vi "Get Block.vi"(8 "error in (no error)":errorcluster, 9 "Remove LenSize? (T)":bool=TRUE, 10 "Block Name":string, 11 "Content in":T2) -> (0 "error out":errorcluster, 1 "Block out":T1, 2 "Data out":string, 3 "Content out":T2, 4 "Found?":bool)   [LabVIEW 2018, in "VI-Hacker.lvlib"]
uses:
  VI-Hacker.lvlib
  TypeDefs/Block.ctl
  TypeDefs/Content.ctl
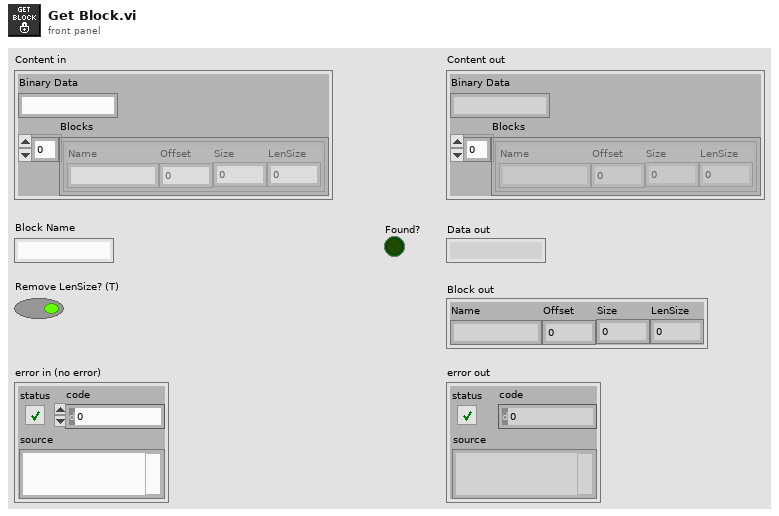
[diagram p1: front panel]
types:
  T1 = typedef "VI-Hacker.lvlib/Block.ctl" = cluster{"Name":string, "Offset":i32, "Size":i32, "LenSize":i32}
  T2 = typedef "VI-Hacker.lvlib/Content.ctl" = cluster{"Binary Data":string, "Blocks":T1[]}
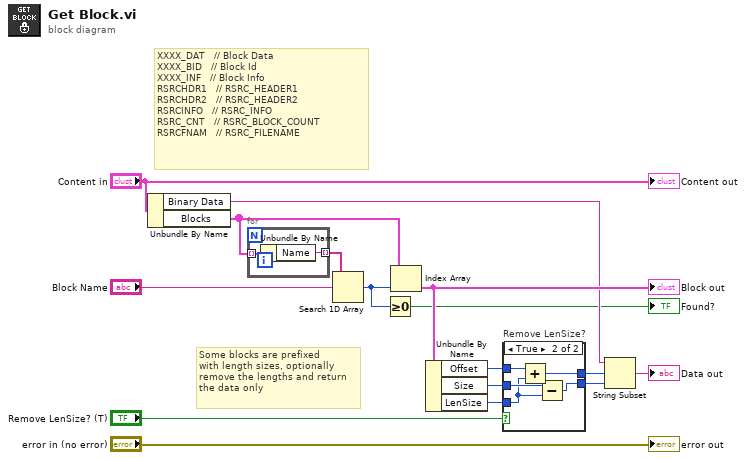
[diagram p0: block diagram]
diagram:
  # "Some blocks are prefixed\nwith length sizes, optionally\nremove the lengths and return\nthe data only"
  # "XXXX_DAT   // Block Data\nXXXX_BID   // Block Id\nXXXX_INF   // Block Info\nRSRCHDR1   // RSRC_HEADER1\nRSRCHDR2   // RSRC_HEADER2\nRSRCINFO   // RSRC_INFO\nRSRC_CNT   // RSRC_BLOCK_COUNT\nRSRCFNAM   // RSRC_FILENAME"
  n1 = Unbundle By Name("Content in") -> ("Binary Data"=w9:string, "Blocks"=w13:T1[])
  n2 = for {
    tunnel: w13 -> [w18] mode=indexing
    tunnel: [w17] -> w14 mode=indexing
    n3 = Unbundle By Name(w18) -> ("Name"=w17:string)
  }
  n4 = Search 1D Array(1D array=w14, element="Block Name") -> (index of element=w2:i32)  [unwired: 1 in]
  n5 = Greater Or Equal To 0?(x=w2) -> (x >= 0?=→"Found?":bool)
  n6 = Index Array(array=w13, index=w2) -> (element=w12:T1)
  "Block out" <- w12
  n7 = Unbundle By Name(w12) -> ("Offset"=w11:i32, "Size"=w10:i32, "LenSize"=w6:i32)
  n8 = case "Remove LenSize?" shown="True" "Remove LenSize? (T)" {
    tunnel: w11 -> [w20 w25]
    tunnel: w10 -> [w19 w24]
    tunnel: [w20 w23] -> w8
    tunnel: [w19 w22] -> w7
    tunnel: w6 -> [_ w21]
    frame False {
    }
    frame True {
      n9 = Add(x=w25, y=w21) -> (x+y=w23:i32)
      n10 = Subtract(x=w24, y=w21) -> (x-y=w22:i32)
    }
  }
  n11 = String Subset(string=w9, offset (0)=w8, length (rest)=w7) -> (substring=→"Data out":string)
  "Content out" <- "Content in"
  "error out" <- "error in (no error)"
